vi "Worked Example--Trapezoidal Rule_ver0.vi"() -> ()   [LabVIEW 2011]
panel:
  out "Approx. Integral":dbl=7.8845418102876925
  out "Waveform Graph":cluster{"Lower limit \"a\"":dbl, dbl, dbl[]}(graph)={"Lower limit \"a\""=0.0, 0.00042, array[10001 elements]}
  in  "Divisions \"N\"":dbl=10000.0
  in  "Upper limit \"b\"":dbl=4.2
  in  "Lower limit \"a\"":dbl
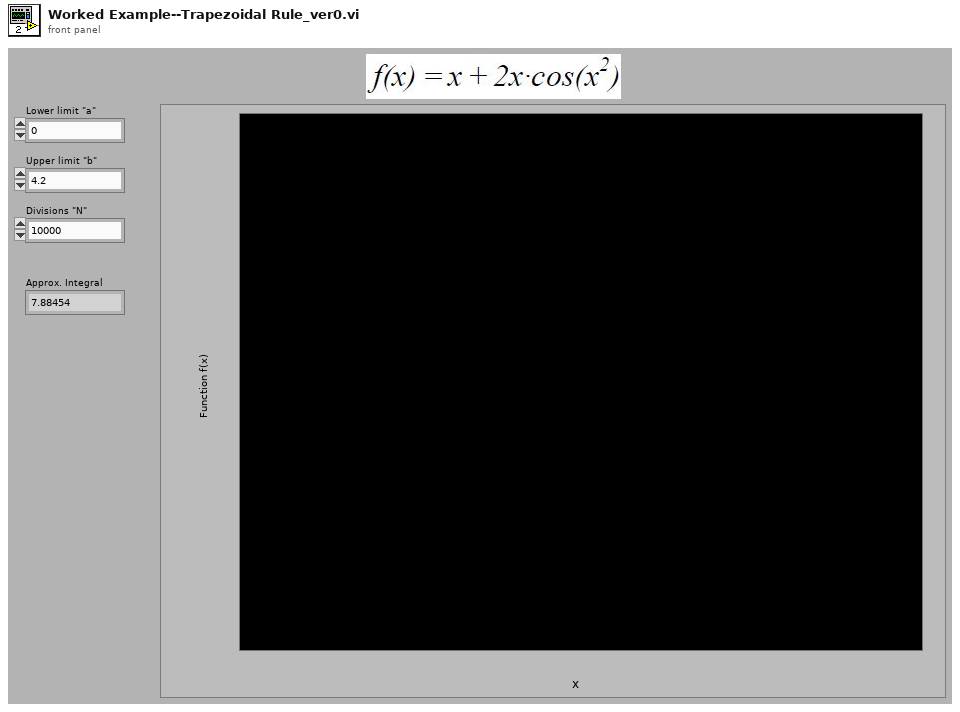
[diagram p1: front panel]
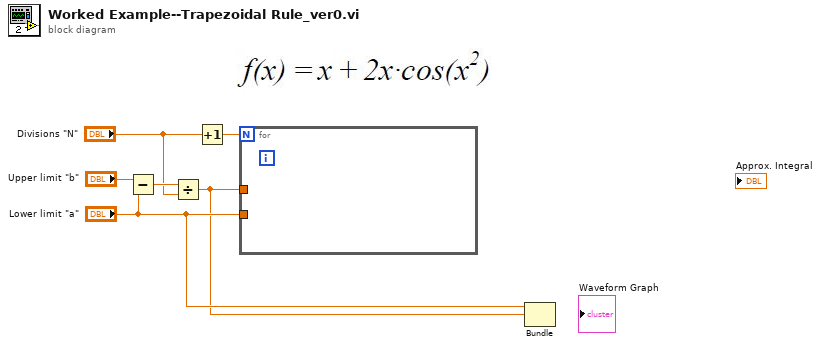
[diagram p0: block diagram]
diagram:
  n1 = Subtract(x="Upper limit \"b\"", y="Lower limit \"a\"") -> (x-y=w5:dbl)
  n2 = Divide(x=w5, y="Divisions \"N\"") -> (x/y=w1:dbl)
  n3 = Increment(x="Divisions \"N\"") -> (x+1=w3:dbl)
  n4 = for {
    N: w3 -> [_]
    tunnel: w1 -> [_]
    tunnel: "Lower limit \"a\"" -> [_]
  }
  n5 = Bundle("Lower limit \"a\""="Lower limit \"a\"", w1) -> ()  [unwired: 2 in, 1 out]
